vi "Get_Paths.vi"(8 "error in (no error)":errorcluster) -> (0 "error out":errorcluster, 2 "Factory_Paths":T1)   [LabVIEW 2020, in "Abstract_Instrument.lvlib" / "Abstract_Instrument.lvclass"]
uses:
  Abstract_Instrument.lvclass
  Typedef/Paths.ctl
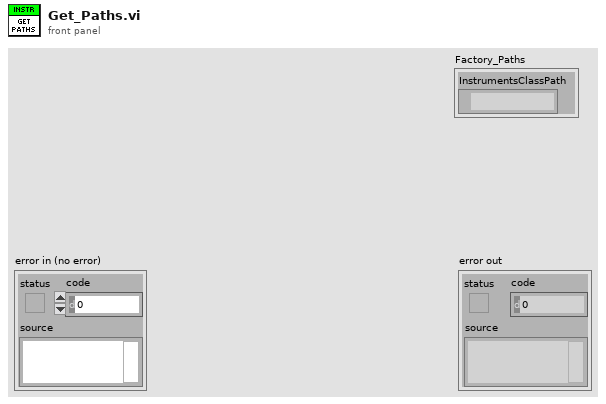
[diagram p1: front panel]
types:
  T1 = typedef "Abstract_Instrument.lvlib/Abstract_Instrument.lvclass/Paths.ctl" = cluster{"InstrumentsClassPath":path}
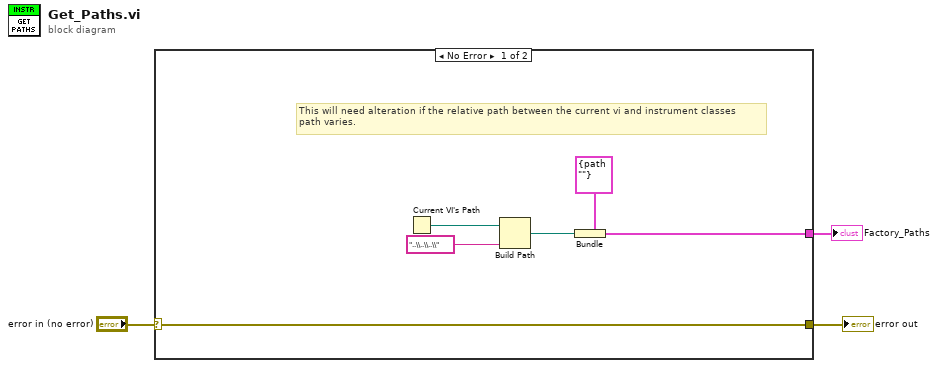
[diagram p0: block diagram]
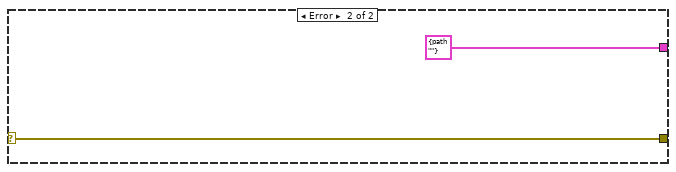
[diagram p2: hidden frame]
diagram:
  n1 = case shown="No Error" "error in (no error)" {
    selector: "error in (no error)" -> [w9 w11]
    tunnel: [w9 w11] -> w2
    tunnel: [w4 T1 {"InstrumentsClassPath"=path ""} ("cluster")] -> w1
    frame No Error {
      # "This will need alteration if the relative path between the current vi and instrument classes\npath varies."
      n2 = Current VI's Path() -> (path=w8:path)
      n3 = Build Path(base path=w8, name or relative path="..\\..\\..\\") -> (appended path=w6:path)
      n4 = Bundle(cluster=T1 {"InstrumentsClassPath"=path ""}, "InstrumentsClassPath"=w6) -> (w4:T1)
    }
    frame Error {
    }
  }
  "error out" <- w2
  "Factory_Paths" <- w1
